vi "File_Handler.vi"(0 "Cans":i32=100, 5 "Cash":T1={"100"=0, "50"=0, "20"=200, "10"=0, "5"=0}, 11 "error in (no error)":errorcluster, 13 "Operations":T2=enum."Write") -> (4 "Cans":i32, 6 "Cash":T1, 15 "error out":errorcluster)   [LabVIEW 2023, in "Vending_machine.lvlib"]
doc: "Handle the writing and retriving of the file data."
uses:
  Vending_machine.lvlib
  Controls/Read_Write.ctl
  Controls/Cash.ctl
  Controls/Denominations.ctl
  <vilib>/Utility/config.llb/Read Key (I32).vi
  <vilib>/Utility/config.llb/Write Key (I32).vi
  <vilib>/Utility/config.llb/NI_LVConfig.lvlib
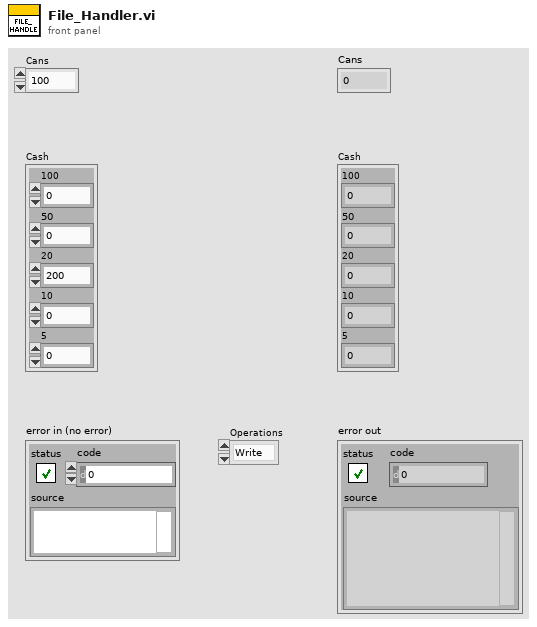
[diagram p1: front panel]
types:
  T1 = typedef "Vending_machine.lvlib/Cash.ctl" = cluster{"100":i32, "50":i32, "20":i32, "10":i32, "5":i32}
  T2 = typedef "Vending_machine.lvlib/Read_Write.ctl" = enum16{"Read", "Write"}
  T3 = typedef "Vending_machine.lvlib/Denominations.ctl" = string[]
  T4 = typedef "NI_LVConfig.lvlib/Config Data RefNum.ctl" = refnum<k1>
  T5 = cluster{"[0]":i32, "[1]":i32, "[2]":i32, "[3]":i32, "[4]":i32}
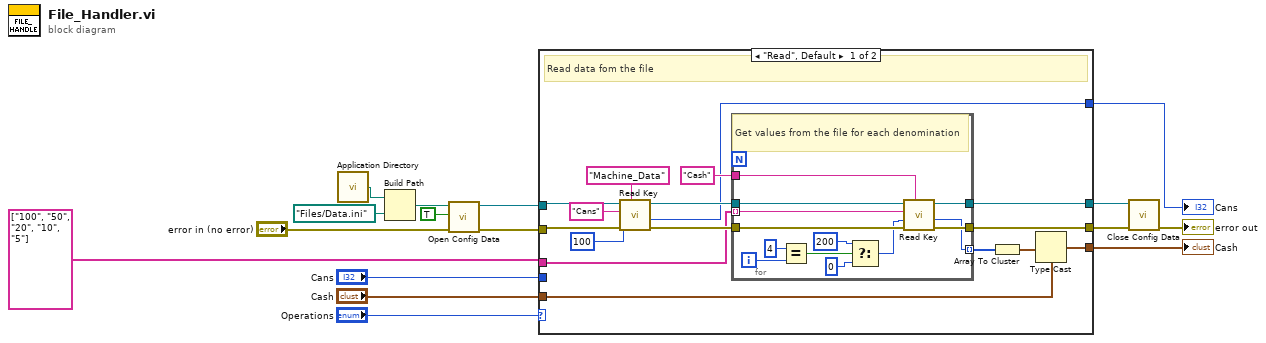
[diagram p0: block diagram]
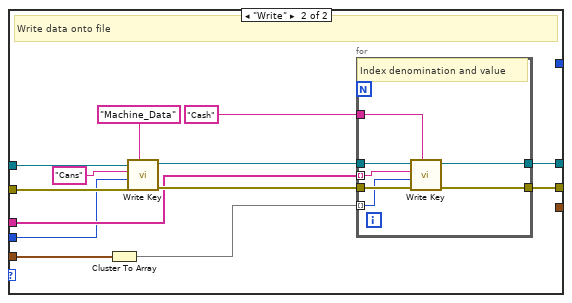
[diagram p2: hidden frame]
diagram:
  n1 = call <vilib>:"Application Directory.vi"() -> ("Application Directory"=w16:path)
  n2 = Build Path(base path=w16, name or relative path=path "Files/Data.ini") -> (appended path=w14:path)
  n3 = call <vilib>:"Open Config Data.vi"("error in (no error)"="error in (no error)", "create file if necessary (T)"=TRUE, "configuration file path"=w14) -> ("error out"=w5:errorcluster, "refnum"=w4:T4)  [unwired: 6 in, 1 out]
  n4 = case shown="\"Read\", Default" "Operations" {
    tunnel: w5 -> [w32 w53]
    tunnel: "Cash" -> [w20 w48]
    tunnel: "Cans" -> [_ w49]
    tunnel: [w27 w52] -> w3
    tunnel: T3 ["100", "50", "20", "10", "5"] -> [w23 w51]
    tunnel: w4 -> [w31 w50]
    tunnel: [w19 _] -> w7
    tunnel: [w18 _] -> w6
    tunnel: [w17 w46] -> w1
    frame "Read", Default {
      # "Read data fom the file"
      n5 = call-poly <vilib>:"Read Key.vi"("section"="Machine_Data", "error in (no error)"=w32, "default value"=100, "key"="Cans", "refnum"=w31) -> ("error out"=w28:errorcluster, "value"=w18:i32, "refnum out"=w24:T4)  [unwired: 3 in, 1 out]
      n6 = for {
        tunnel: w28 -> [w45]
        tunnel: "Cash" ("section") -> [w44]
        tunnel: [w43] -> w27
        tunnel: [w42] -> w17
        tunnel: w24 -> [w41]
        tunnel: w23 -> [w40] mode=indexing
        tunnel: [w33] -> w22 mode=indexing
        i -> [w39]
        # "Get values from the file for each denomination"
        n7 = Equal?(x=4, y=w39) -> (x = y?=w37:bool)
        n8 = Select(t=200 ("x"), s=w37, f=0 ("x")) -> (s? t:f=w34:i32)
        n9 = call-poly <vilib>:"Read Key.vi"("section"=w44, "error in (no error)"=w45, "default value"=w34, "key"=w40, "refnum"=w41) -> ("error out"=w43:errorcluster, "value"=w33:i32, "refnum out"=w42:T4)  [unwired: 3 in, 1 out]
      }
      n10 = Array To Cluster(array=w22) -> (cluster=w21:T5)
      n11 = Type Cast(type=w20, x=w21) -> (*(type *) &x=w19:T1)
    }
    frame "Write" {
      # "Write data onto file"
      n12 = Cluster To Array(cluster=w48) -> (array=w47:i32[])
      n13 = call-poly <vilib>:"Write Key.vi"("section"="Machine_Data", "error in (no error)"=w53, "value"=w49, "key"="Cans", "refnum"=w50) -> ("error out"=w56:errorcluster, "refnum out"=w55:T4)  [unwired: 4 in, 1 out]
      n14 = for {
        tunnel: w55 -> [w65]
        tunnel: w56 -> [w64]
        tunnel: "Cash" ("section") -> [w63]
        tunnel: [w62] -> w52
        tunnel: w51 -> [w61] mode=indexing
        tunnel: w47 -> [w60] mode=indexing
        tunnel: [w59] -> w46
        # "Index denomination and value"
        n15 = call-poly <vilib>:"Write Key.vi"("section"=w63, "error in (no error)"=w64, "value"=w60, "key"=w61, "refnum"=w65) -> ("error out"=w62:errorcluster, "refnum out"=w59:T4)  [unwired: 4 in, 1 out]
      }
    }
  }
  "Cash" <- w7
  "Cans" <- w6
  n16 = call <vilib>:"Close Config Data.vi"("error in (no error)"=w3, "refnum"=w1) -> ("error out"=→"error out":errorcluster)  [unwired: 8 in, 1 out]
